vi "magnetic-actuator-safe-copy.vi"() -> ()   [LabVIEW 2024]
uses:
  mag-settings.ctl
panel:
  in  "Reflux Ratio":bool
  in  "Total Withdrawl":bool
  in  "Total Reflux":bool
  in  "On":bool
  in  "Off":bool
  out "Cycle Running":bool
  out "Last Command Sent":string
  out "Countdown Timer (mS)":u32
  out "last event":u32
  out "Coil Active":bool
  in  "Stop Cycle":bool
  in  "Start Cycle":bool
  in  "Eng Mode":bool
  out "LOW Cycle Time (Seconds)":dbl
  out "HIGH Cycle Time (Seconds)":dbl
  out "Duty %":dbl
  in  "Reflux Ratio":dbl
  in  "Period (Seconds)":dbl=5.0
  in  "Exit Program":bool
  # "Time On = 0 (aways off)"
  # "Time On = 1 (aways on)"
  # "TODO: MAKE THIS AESTHETIC"
  # "HIGH Cycle = period*(1/1+Reflux Ratio)"
  # "LOW Cycle = period - HIGH Cycle Time"
  # "Manual Controls"
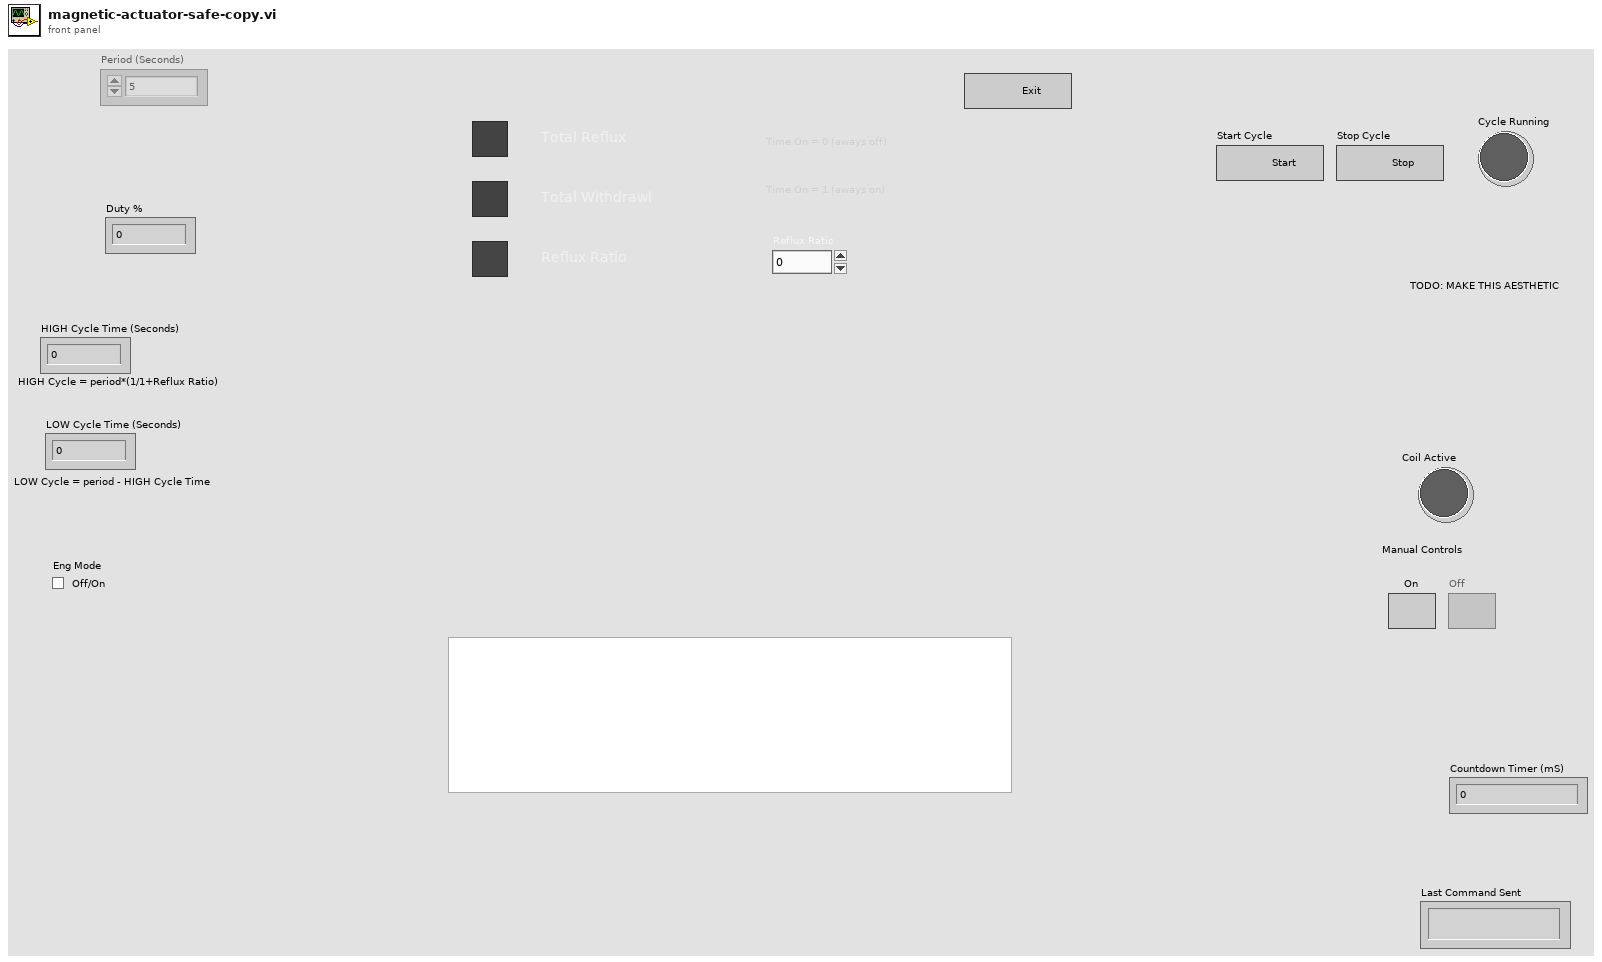
[diagram p1: front panel]
types:
  T1 = typedef "mag-settings.ctl" = cluster{"COM Port (COM10)":refnum<visa-resource-name>, "ADAM-ID":dbl, "ADAM-DO-channel":dbl, "Period (Seconds)":dbl, "Duty Cycle":dbl, "Eng Mode":bool}
  T2 = enum8{"Enabled", "Disabled", "Disabled and Grayed Out"}
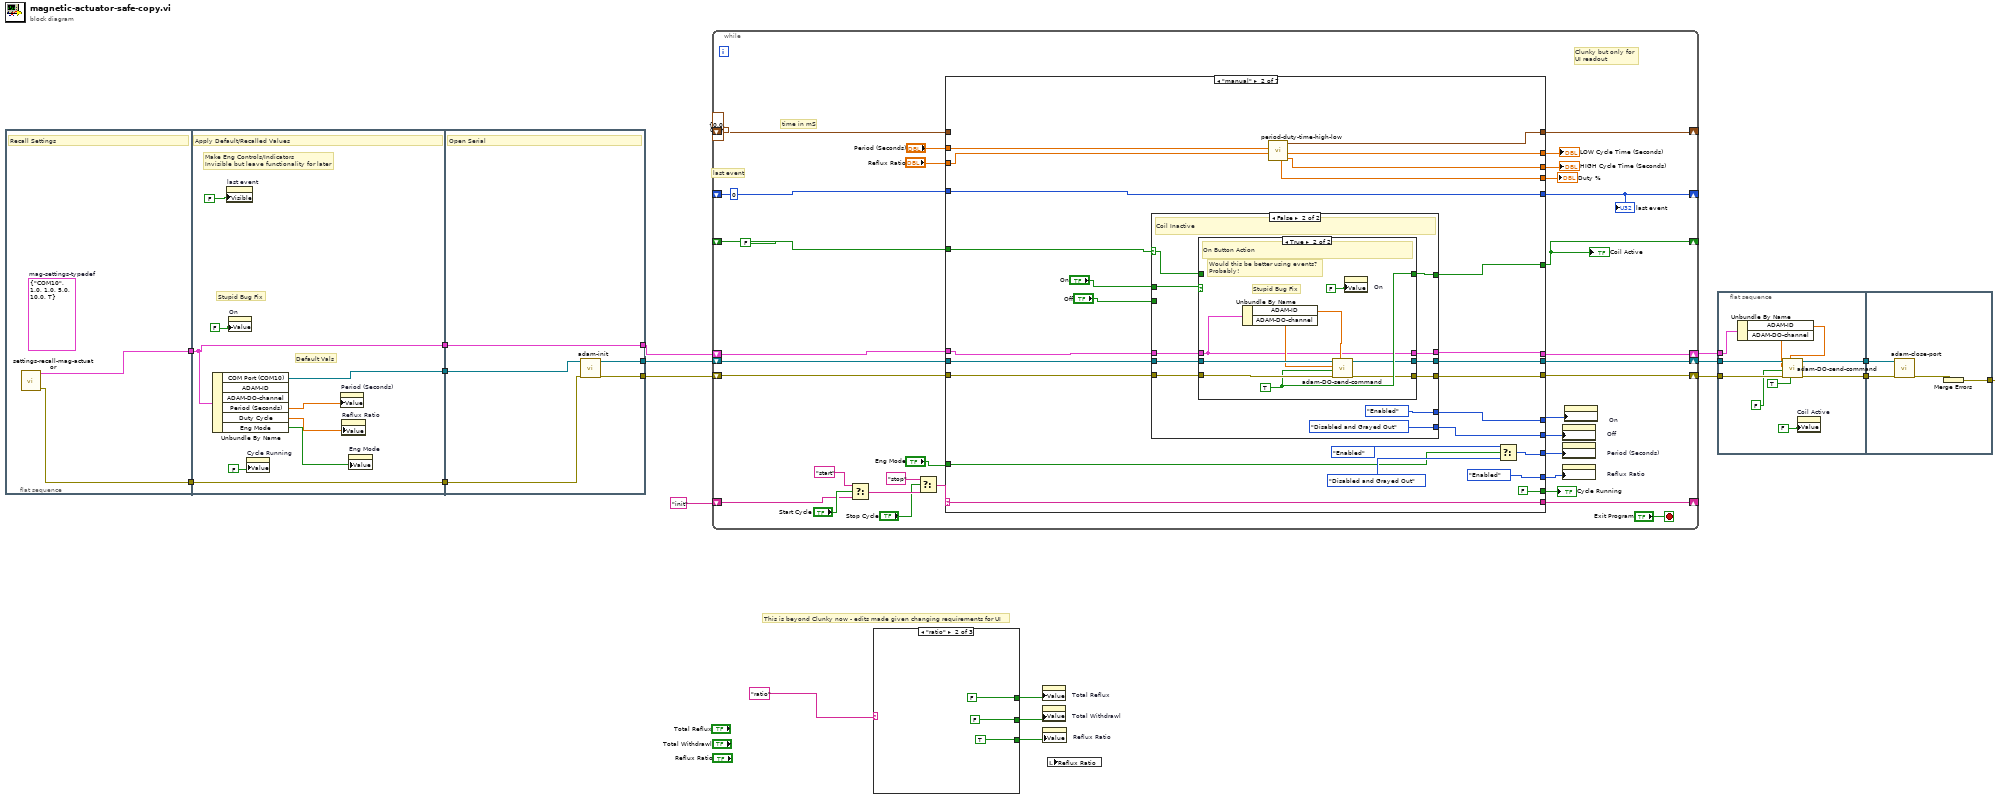
[diagram p0: block diagram]
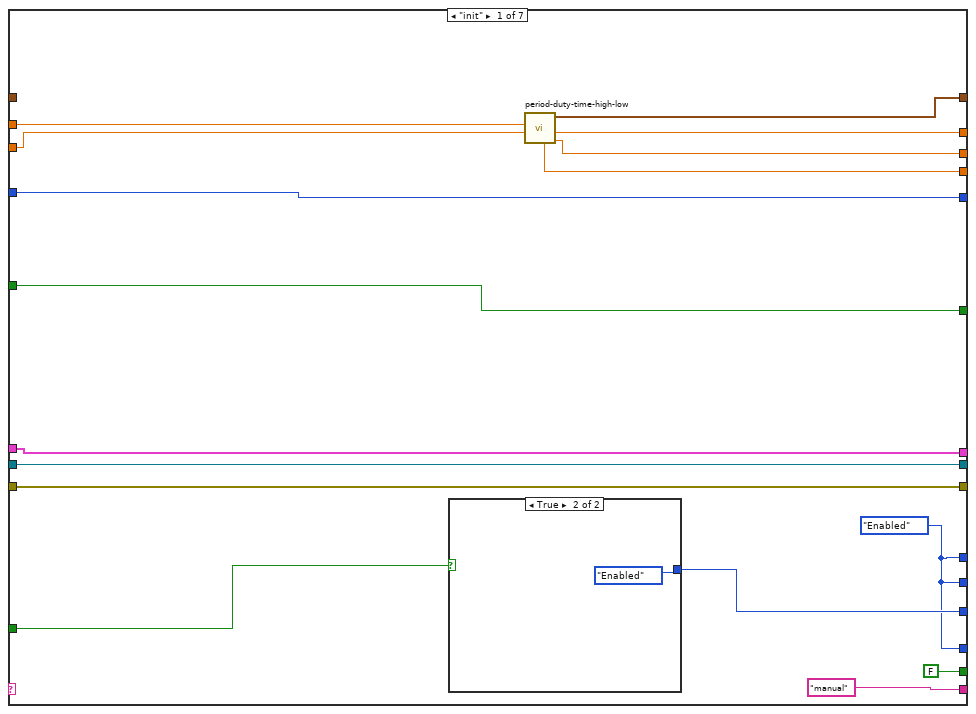
[diagram p4: hidden frame]
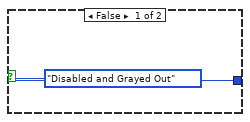
[diagram p5: hidden frame]
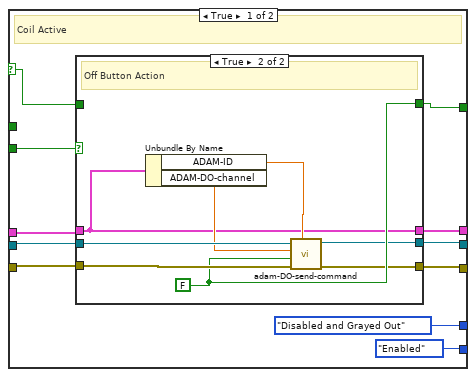
[diagram p6: hidden frame]
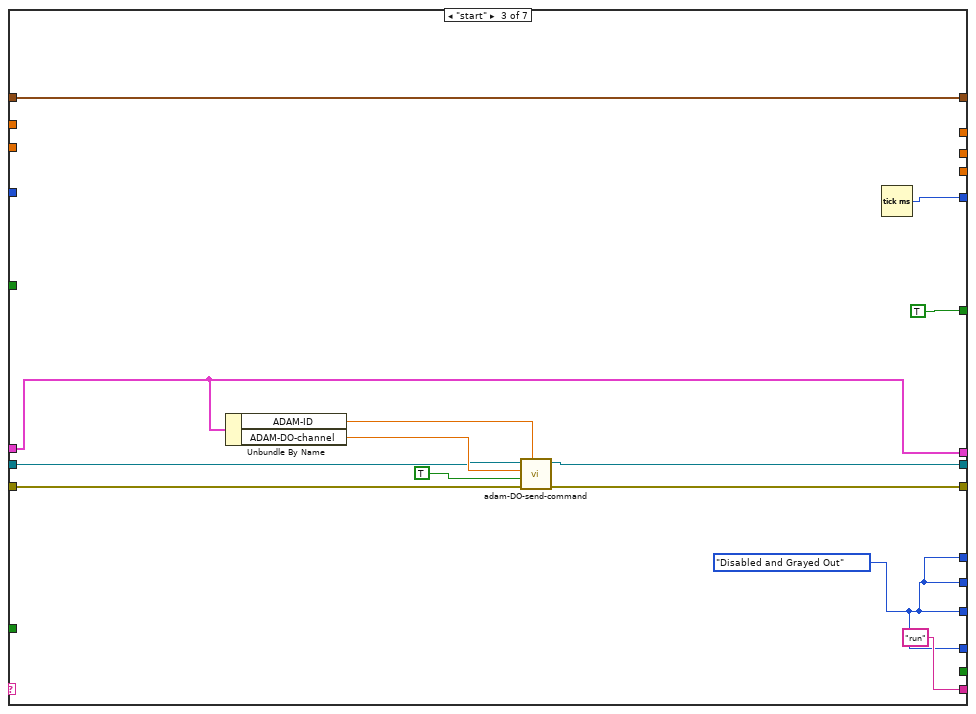
[diagram p9: hidden frame]
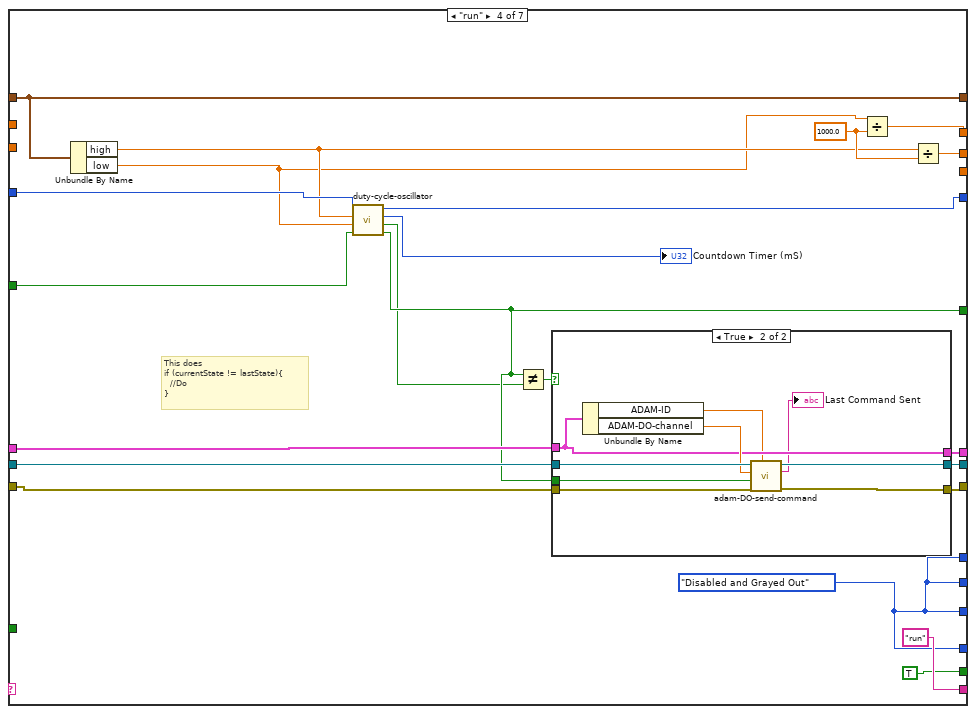
[diagram p10: hidden frame]
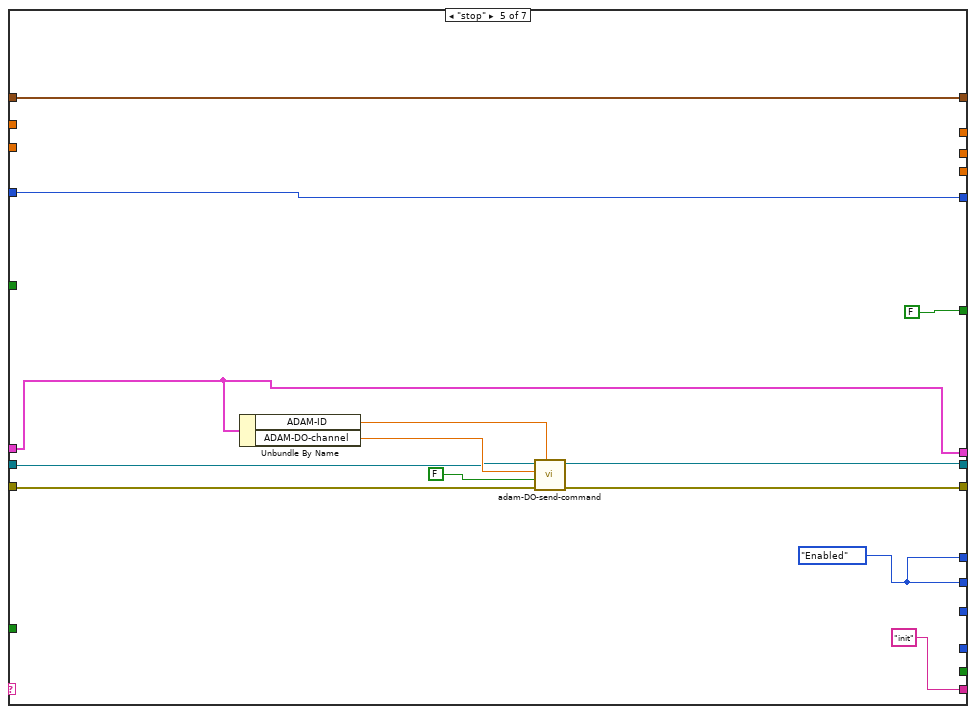
[diagram p12: hidden frame]
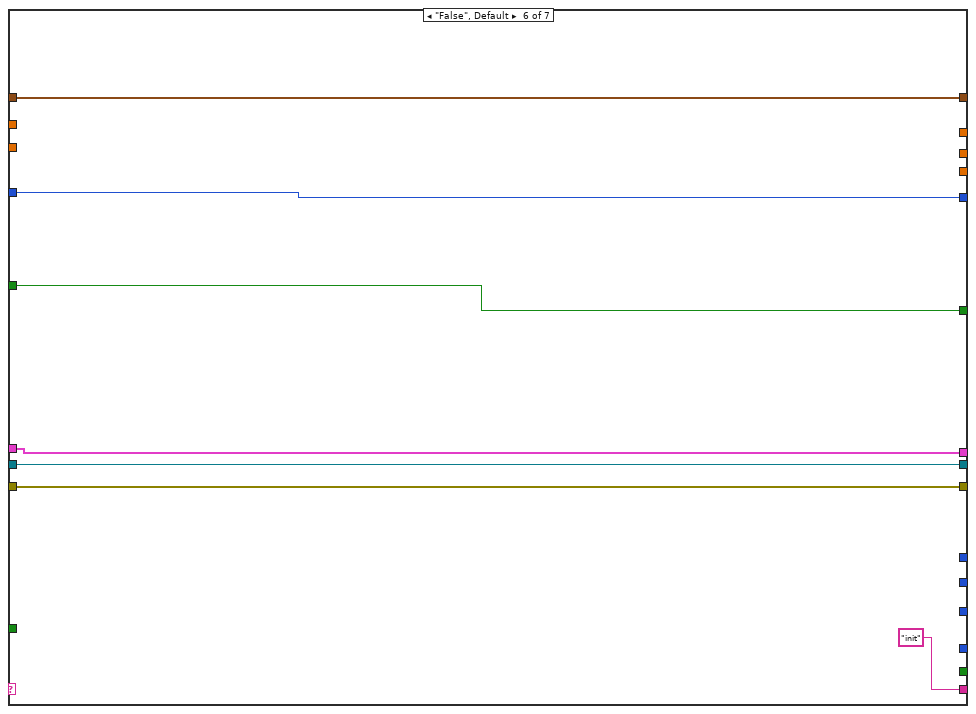
[diagram p13: hidden frame]
diagram:
  # "This is beyond Clunky now - edits made given changing requirements for UI"
  # "last event"
  n1 = flat-sequence {
    tunnel: [w23] -> w19
    tunnel: [w22] -> w11
    tunnel: [w32] -> w20
    tunnel: w19 -> [w31]
    tunnel: [w31] -> w18
    tunnel: w11 -> [w30]
    tunnel: [w30] -> w10
    tunnel: [w37] -> w17
    tunnel: [w36] -> w16
    tunnel: w20 -> [w34]
    tunnel: w18 -> [w35]
    tunnel: [w33] -> w9
    tunnel: w10 -> [w33]
    frame #0 {
      (unwired) T1 {"COM Port (COM10)"="COM10", "ADAM-ID"=1.0, "ADAM-DO-channel"=1.0, "Period (Seconds)"=5.0, "Duty Cycle"=10.0, "Eng Mode"=TRUE}  # mag-settings-typedef
      # "Recall Settings"
      n2 = call "settings-recall-mag-actuator.vi"() -> ("error out"=w23:errorcluster, "mag-settings"=w22:T1)  [unwired: 9 in, 1 out]
    }
    frame #1 {
      # "Default Vals"
      # "Make Eng Controls/Indicators\nInvisible but leave functionality for later"
      # "Stupid Bug Fix"
      # "Apply Default/Recalled Values"
      n3 = Unbundle By Name(w30) -> ("COM Port (COM10)"=w32:refnum<visa-resource-name>, "Period (Seconds)"=w29:dbl, "Duty Cycle"=w28:dbl, "Eng Mode"=w27:bool)  [unwired: 2 out]
      n4 = property on="last event" class="DigNum (strict)"("Visible"=FALSE) -> ()  [unwired: 2 in, 2 out]
      n5 = property on="On" class="Bool (strict)"("Value"=FALSE ("On")) -> ()  [unwired: 2 in, 2 out]
      n6 = property on="Cycle Running" class="Bool (strict)"("Value"=FALSE ("Running")) -> ()  [unwired: 2 in, 2 out]
      n7 = property on="Period (Seconds)" class="DigNum (strict)"("Value"=w29) -> ()  [unwired: 2 in, 2 out]
      n8 = property on="Reflux Ratio" class="DigNum (strict)"("Value"=w28) -> ()  [unwired: 2 in, 2 out]
      n9 = property on="Eng Mode" class="Bool (strict)"("Value"=w27) -> ()  [unwired: 2 in, 2 out]
    }
    frame #2 {
      # "Open Serial"
      n10 = call "adam-init.vi"("error in (no error)"=w35, "COM Port (COM10)"=w34) -> ("error out"=w36:errorcluster, "VISA resource name out"=w37:refnum<visa-resource-name>)  [unwired: 8 in]
    }
  }
  n11 = while {
    shift-right: [w63] -> _
    shift-left: "init" -> [w43]
    shift-right: [w62] -> _
    shift-left: u32 0 ("millisecond timer value") -> [w61]
    shift-right: [w41] -> _
    shift-left: cluster{"low":dbl, "high":dbl} {"low"=0.0, "high"=0.0} ("delaytimes mS") -> [w60]
    shift-right: [w57] -> _
    shift-left: FALSE ("t") -> [w56]
    shift-right: [w53] -> w13
    shift-left: w17 -> [w52]
    shift-right: [w51] -> w12
    shift-left: w16 -> [w50]
    shift-right: [w48] -> w8
    shift-left: w9 -> [w49]
    stop <- "Exit Program" stop-if-true
    # "time in mS"
    # "Clunky but only for\nUI readout"
    n12 = Select(t="start", s="Start Cycle", f=w43) -> (s? t:f=w55:string)
    n13 = Select(t="stop", s="Stop Cycle", f=w55) -> (s? t:f=w66:string)
    n14 = case shown="\"manual\"" w66 {
      selector: w66 -> [_ w113 _ _ _ _ w231]
      tunnel: "Period (Seconds)" -> [w80 w111 _ _ _ _ _]
      tunnel: ["manual" w113 "run" "run" "init" "init" w231] -> w63
      tunnel: [w78 w109 w172 w194 w218 w227 w233] -> w62
      tunnel: w61 -> [w78 w109 _ w179 w218 w227 w233]
      tunnel: [w81 w112 w171 w188 w217 w226 w234] -> w41
      tunnel: w60 -> [_ _ w171 w188 w217 w226 w234]
      tunnel: [w84 w103 w161 w184 _ _ _] -> w59
      tunnel: "Eng Mode" -> [w85 w100 _ _ _ _ _]
      tunnel: [w70 T2."Enabled" ("Disabled") w161 w184 _ _ _] -> w58
      tunnel: [w75 w96 TRUE ("t") w181 FALSE ("t") w221 w232] -> w57
      tunnel: w56 -> [w75 w106 _ w182 _ w221 w232]
      tunnel: [w83 w95 w163 w192 w210 w224 w230] -> w53
      tunnel: w52 -> [w83 w97 w164 w191 w211 w224 w230]
      tunnel: [w82 w94 w162 w190 w209 w223 w229] -> w51
      tunnel: w50 -> [w82 w99 w168 w189 w212 w223 w229]
      tunnel: "Reflux Ratio" -> [w79 w110 _ _ _ _ _]
      tunnel: w49 -> [w77 w98 w169 w187 w213 w222 w228]
      tunnel: [w77 w93 w169 w186 w213 w222 w228] -> w48
      tunnel: [FALSE ("Running") FALSE ("Running") _ TRUE ("Running") _ _ _] -> w47
      tunnel: [w70 w105 w161 w184 w208 _ _] -> w46
      tunnel: [w70 w104 w161 w184 w208 _ _] -> w45
      tunnel: [w73 w92 _ w178 _ _ _] -> w40
      tunnel: [w72 w91 _ w177 _ _ _] -> w39
      tunnel: [w71 w90 _ _ _ _ _] -> w42
      frame "init" {
        w70 = T2."Enabled" ("Disabled")
        n15 = case shown="True" w85 {
          tunnel: [T2."Disabled and Grayed Out" ("Disabled") T2."Enabled" ("Disabled")] -> w84
          frame False {
          }
          frame True {
          }
        }
        n16 = call "period-duty-time-high-low.vi"("Duty Cycle"=w79, "Period (Seconds)"=w80) -> ("Time High (Seconds)"=w72:dbl, "Time Low (Seconds)"=w73:dbl, "delaytimes mS"=w81:cluster{"low":dbl, "high":dbl}, "Duty %"=w71:dbl)  [unwired: 6 in]
      }
      frame "manual" {
        n17 = case shown="False" w106 {
          selector: w106 -> [w121 w138]
          tunnel: [T2."Enabled" ("Disabled") T2."Disabled and Grayed Out" ("Disabled")] -> w105
          tunnel: [T2."Disabled and Grayed Out" ("Disabled") T2."Enabled" ("Disabled")] -> w104
          tunnel: "On" -> [_ w145]
          tunnel: w99 -> [w116 w144]
          tunnel: w98 -> [w115 w143]
          tunnel: w97 -> [w117 w142]
          tunnel: [w120 w141] -> w96
          tunnel: [w119 w140] -> w95
          tunnel: [w118 w139] -> w94
          tunnel: "Off" -> [w122 _]
          tunnel: [w114 w137] -> w93
          frame True {
            # "Coil Active"
            n18 = case shown="True" w122 {
              tunnel: w116 -> [w125 w136]
              tunnel: w115 -> [w127 w129]
              tunnel: w117 -> [w126 w135]
              tunnel: [w128 w134] -> w120
              tunnel: [w126 w133] -> w119
              tunnel: [w125 w132] -> w118
              tunnel: w121 -> [w128 _]
              tunnel: [w127 w129] -> w114
              frame False {
              }
              frame True {
                w134 = FALSE ("Channel Active")
                # "Off Button Action"
                n19 = Unbundle By Name(w129) -> ("ADAM-ID"=w131:dbl, "ADAM-DO-channel"=w130:dbl)
                n20 = call "adam-DO-send-command.vi"("Device Address"=w131, "error in (no error)"=w136, "Channel Active"=w134, "Channel Number"=w130, "VISA Refnum in"=w135) -> ("error out"=w132:errorcluster, "VISA Refnum out"=w133:refnum<visa-resource-name>)  [unwired: 1 in, 4 out]
              }
            }
          }
          frame False {
            # "Coil Inactive"
            n21 = case shown="True" w145 {
              tunnel: w144 -> [w148 w160]
              tunnel: w143 -> [w150 w153]
              tunnel: w142 -> [w149 w159]
              tunnel: [w151 w158] -> w141
              tunnel: [w149 w157] -> w140
              tunnel: [w148 w156] -> w139
              tunnel: w138 -> [w151 _]
              tunnel: [w150 w153] -> w137
              frame False {
              }
              frame True {
                w158 = TRUE ("Channel Active")
                # "Stupid Bug Fix"
                # "Would this be better using events?\nProbably!"
                # "On Button Action"
                n22 = Unbundle By Name(w153) -> ("ADAM-ID"=w155:dbl, "ADAM-DO-channel"=w154:dbl)
                n23 = call "adam-DO-send-command.vi"("Device Address"=w155, "error in (no error)"=w160, "Channel Active"=w158, "Channel Number"=w154, "VISA Refnum in"=w159) -> ("error out"=w156:errorcluster, "VISA Refnum out"=w157:refnum<visa-resource-name>)  [unwired: 1 in, 4 out]
                n24 = property on="On" class="Bool (strict)"("Value"=FALSE ("On")) -> ()  [unwired: 2 in, 2 out]
              }
            }
          }
        }
        n25 = call "period-duty-time-high-low.vi"("Duty Cycle"=w110, "Period (Seconds)"=w111) -> ("Time High (Seconds)"=w91:dbl, "Time Low (Seconds)"=w92:dbl, "delaytimes mS"=w112:cluster{"low":dbl, "high":dbl}, "Duty %"=w90:dbl)  [unwired: 6 in]
        n26 = Select(t=T2."Enabled" ("Disabled"), s=w100, f=T2."Disabled and Grayed Out" ("Disabled")) -> (s? t:f=w103:T2)
      }
      frame "start" {
        w161 = T2."Disabled and Grayed Out" ("Disabled")
        n27 = Unbundle By Name(w169) -> ("ADAM-ID"=w166:dbl, "ADAM-DO-channel"=w167:dbl)
        n28 = call "adam-DO-send-command.vi"("Device Address"=w166, "error in (no error)"=w168, "Channel Active"=TRUE, "Channel Number"=w167, "VISA Refnum in"=w164) -> ("error out"=w162:errorcluster, "VISA Refnum out"=w163:refnum<visa-resource-name>)  [unwired: 1 in, 4 out]
        n29 = Tick Count (ms)() -> (millisecond timer value=w172:u32)
      }
      frame "run" {
        w176 = 1000.0 ("y")
        w184 = T2."Disabled and Grayed Out" ("Disabled")
        # "This does\nif (currentState != lastState){\n  //Do\n}"
        n30 = Unbundle By Name(w188) -> ("high"=w175:dbl, "low"=w174:dbl)
        n31 = call "duty-cycle-oscillator.vi"("Input State"=w182, "time low mS"=w174, "time high mS"=w175, "lastEvent mS"=w179) -> ("output state"=w181:bool, "lastState"=w180:bool, "Countdown Timer (mS)"=→"Countdown Timer (mS)":u32, "lastEvent ms Out"=w194:u32)  [unwired: 4 in]
        n32 = Not Equal?(x=w181, y=w180) -> (x != y?=w193:bool)
        n33 = case shown="True" w193 {
          tunnel: [w198 w204] -> w192
          tunnel: w191 -> [w198 w206]
          tunnel: [w197 w203] -> w190
          tunnel: w189 -> [w197 w205]
          tunnel: w187 -> [w196 w201]
          tunnel: [w196 w201] -> w186
          tunnel: w181 -> [_ w207]
          frame False {
          }
          frame True {
            n34 = Unbundle By Name(w201) -> ("ADAM-ID"=w200:dbl, "ADAM-DO-channel"=w202:dbl)
            n35 = call "adam-DO-send-command.vi"("Device Address"=w200, "error in (no error)"=w205, "Channel Active"=w207, "Channel Number"=w202, "VISA Refnum in"=w206) -> ("error out"=w203:errorcluster, "command"=→"Last Command Sent":string, "VISA Refnum out"=w204:refnum<visa-resource-name>)  [unwired: 1 in, 3 out]
          }
        }
        n36 = Divide(x=w174, y=w176) -> (x/y=w178:dbl)
        n37 = Divide(x=w175, y=w176) -> (x/y=w177:dbl)
      }
      frame "stop" {
        w208 = T2."Enabled" ("Disabled")
        n38 = Unbundle By Name(w213) -> ("ADAM-ID"=w215:dbl, "ADAM-DO-channel"=w216:dbl)
        n39 = call "adam-DO-send-command.vi"("Device Address"=w215, "error in (no error)"=w212, "Channel Active"=FALSE, "Channel Number"=w216, "VISA Refnum in"=w211) -> ("error out"=w209:errorcluster, "VISA Refnum out"=w210:refnum<visa-resource-name>)  [unwired: 1 in, 4 out]
      }
      frame "False", Default {
      }
      frame "True" {
      }
    }
    "Coil Active" <- w57
    "last event" <- w62
    "Cycle Running" <- w47
    "Duty %" <- w42
    "HIGH Cycle Time (Seconds)" <- w39
    "LOW Cycle Time (Seconds)" <- w40
    n40 = property on="Off" class="Bool"("DisabledEnum"=w46) -> ()  [unwired: 2 in, 2 out]
    n41 = property on="Period (Seconds)" class="DigNum (strict)"("DisabledEnum"=w59) -> ()  [unwired: 2 in, 2 out]
    n42 = property on="Reflux Ratio" class="DigNum (strict)"("DisabledEnum"=w58) -> ()  [unwired: 2 in, 2 out]
    n43 = property on="On" class="Bool (strict)"("DisabledEnum"=w45) -> ()  [unwired: 2 in, 2 out]
  }
  n44 = case shown="\"ratio\"" "ratio" {
    tunnel: [_ FALSE ("Total Reflux") _] -> w4
    tunnel: [_ FALSE ("Total Withdrawl") _] -> w3
    tunnel: [_ TRUE ("Reflux Ratio") _] -> w2
    frame "False", Default {
    }
    frame "ratio" {
    }
    frame "True" {
      # "User Mode"
    }
  }
  n45 = property on="Total Reflux" class="Bool (strict)"("Value"=w4) -> ()  [unwired: 2 in, 2 out]
  n46 = property on="Total Withdrawl" class="Bool (strict)"("Value"=w3) -> ()  [unwired: 2 in, 2 out]
  n47 = property on="Reflux Ratio" class="Bool (strict)"("Value"=w2) -> ()  [unwired: 2 in, 2 out]
  n48 = local read "Reflux Ratio"() -> ()  [unwired: 1 in]
  n49 = flat-sequence {
    tunnel: w12 -> [w247]
    tunnel: w13 -> [w243]
    tunnel: [w246] -> w15
    tunnel: [w244] -> w14
    tunnel: w8 -> [w241]
    tunnel: w15 -> [w249]
    tunnel: w14 -> [w250]
    tunnel: [w248] -> _
    frame #0 {
      n50 = Unbundle By Name(w241) -> ("ADAM-ID"=w239:dbl, "ADAM-DO-channel"=w240:dbl)
      n51 = call "adam-DO-send-command.vi"("Stop All"=TRUE, "Device Address"=w239, "error in (no error)"=w247, "Channel Active"=FALSE, "Channel Number"=w240, "VISA Refnum in"=w243) -> ("error out"=w244:errorcluster, "VISA Refnum out"=w246:refnum<visa-resource-name>)  [unwired: 4 out]
      n52 = property on="Coil Active" class="Bool (strict)"("Value"=FALSE ("Coil Active")) -> ()  [unwired: 2 in, 2 out]
    }
    frame #1 {
      n53 = call "adam-close-port.vi"("error in (no error)"=w250, "VISA Refnum in"=w249) -> ("error out"=w251:errorcluster)  [unwired: 9 in]
      n54 = Merge Errors(w251) -> (w248:errorcluster)
    }
  }
